vi "doRabi.vi"(8 "q_samples":i32=50, 9 "MW_Parameters":T1, 10 "parameters_recenter":T4={"input_xyz"={"X_um"=0.0, "Y_um"=0.0, "Z_um"=0.0}, "recenter"=FALSE, "recenter_s"=3}, 11 "Rabi_parameters":T5) -> (0 "triggers":u32[][](array[numeric]), 1 "std_deviation":dbl[](array[numeric]), 2 "Rabi_curve":cluster{dbl[], "dark_time_us":dbl[]}(graph), 3 "timetags":u32[][](array[numeric]))   [LabVIEW 2018]
uses:
  <vilib>/Analysis/NI_AALBase.lvlib
  <instrlib>/Rohde&Schwarz RF Signal Generator/Rohde&Schwarz RF Signal Generator.lvlib
panel:
  in  "parameters_z-scan":T2={"dwell_time_ms"=2.0, "q_steps"=5, "span_um"=1.0, "refocus"=TRUE}
  in  "parameters_xy-scan":T3={"image_size_xy_um"=2.0, "frame_size_xy_px"=7, "dwell_time_ms"=0.5}
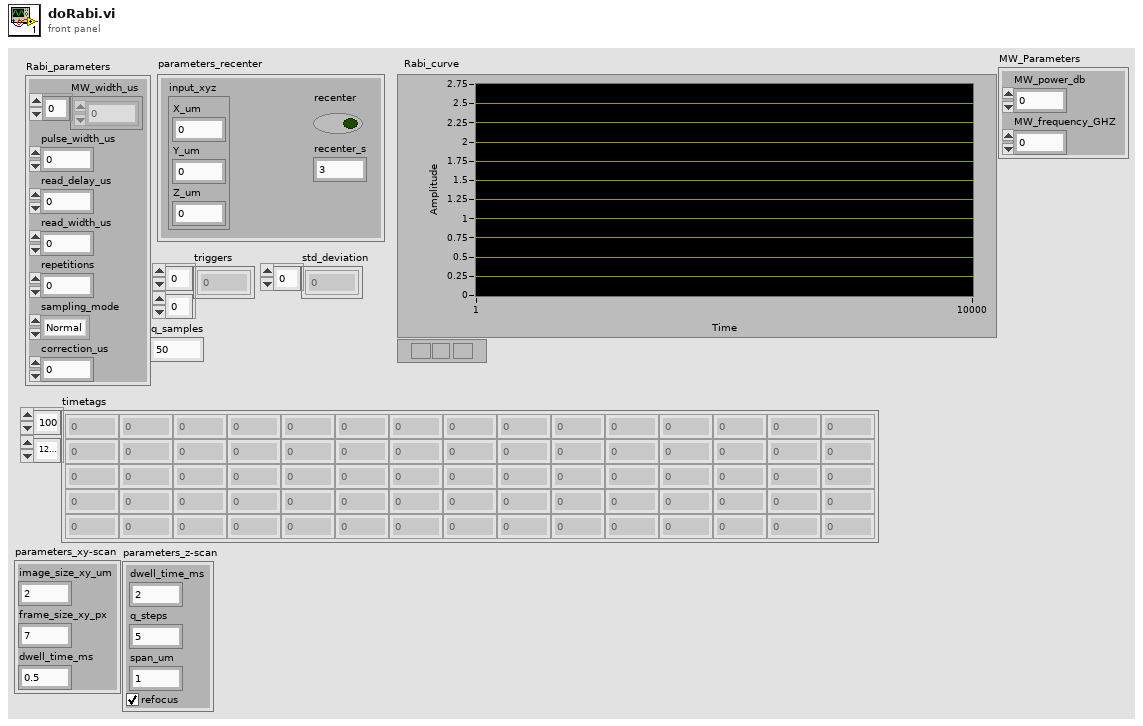
[diagram p1: front panel]
types:
  T1 = cluster{"MW_power_db":dbl, "MW_frequency_GHZ":dbl}
  T2 = cluster{"dwell_time_ms":dbl, "q_steps":u32, "span_um":dbl, "refocus":bool}
  T3 = cluster{"image_size_xy_um":dbl, "frame_size_xy_px":u32, "dwell_time_ms":dbl}
  T4 = cluster{"input_xyz":cluster{"X_um":sgl, "Y_um":sgl, "Z_um":sgl}, "recenter":bool, "recenter_s":u32}
  T5 = cluster{"MW_width_us":dbl[], "pulse_width_us":dbl, "read_delay_us":dbl, "read_width_us":dbl, "repetitions":i32, "sampling_mode":enum16{"Normal", "Sweep"}, "correction_us":dbl}
  T6 = cluster{"file_path":path, "file_name":string, "image":dbl[][][], "image_size_xy":cluster{"image_size_x_um":sgl, "image_size_y_um":sgl}, "pixel_dwell_time_ms":sgl, "Laser_power_mW":sgl, "pixel_size":dbl, "tile_ij":cluster{"tile_i":i32, "tile_j":i32}, "Objective":string, "ColorMarkers":cluster{dbl, u32}[], "timestamp":timestamp, "micro-position-xyz":cluster{"micro-position_x_mm":sgl, "micro-position_y_mm":sgl, "micro-position_z_mm":sgl}, "zero_xyz":cluster{"zero_x_mm":dbl, "zero_y_mm":dbl, "zero_z_mm":dbl}, "nano-position-xyz":cluster{"nano-position_x_V":sgl, "nano-position_y_V":sgl, "nano-position_z_V":sgl}, "Kxyz":cluster{"Kx_V/um":sgl, "Ky_V/um":sgl, "Kz_V/um":sgl}}
  T7 = cluster{"x_um":sgl[], "y_um":sgl[], "z_um":sgl[], "timetag":timestamp[]}
  T8 = cluster{"Instruct Data":i32, "Op Code":i32, "Flags":bool[], "Comments":string, "Time":dbl}[]
  T9 = cluster{"nano-position_X_um":sgl, "nano-position_Y_um":sgl, "nano-position Z_um":sgl}
  T10 = cluster{"nano-position_X_um":sgl, "nano-position_Y_um":sgl, "nano-position Z_um":sgl}[]
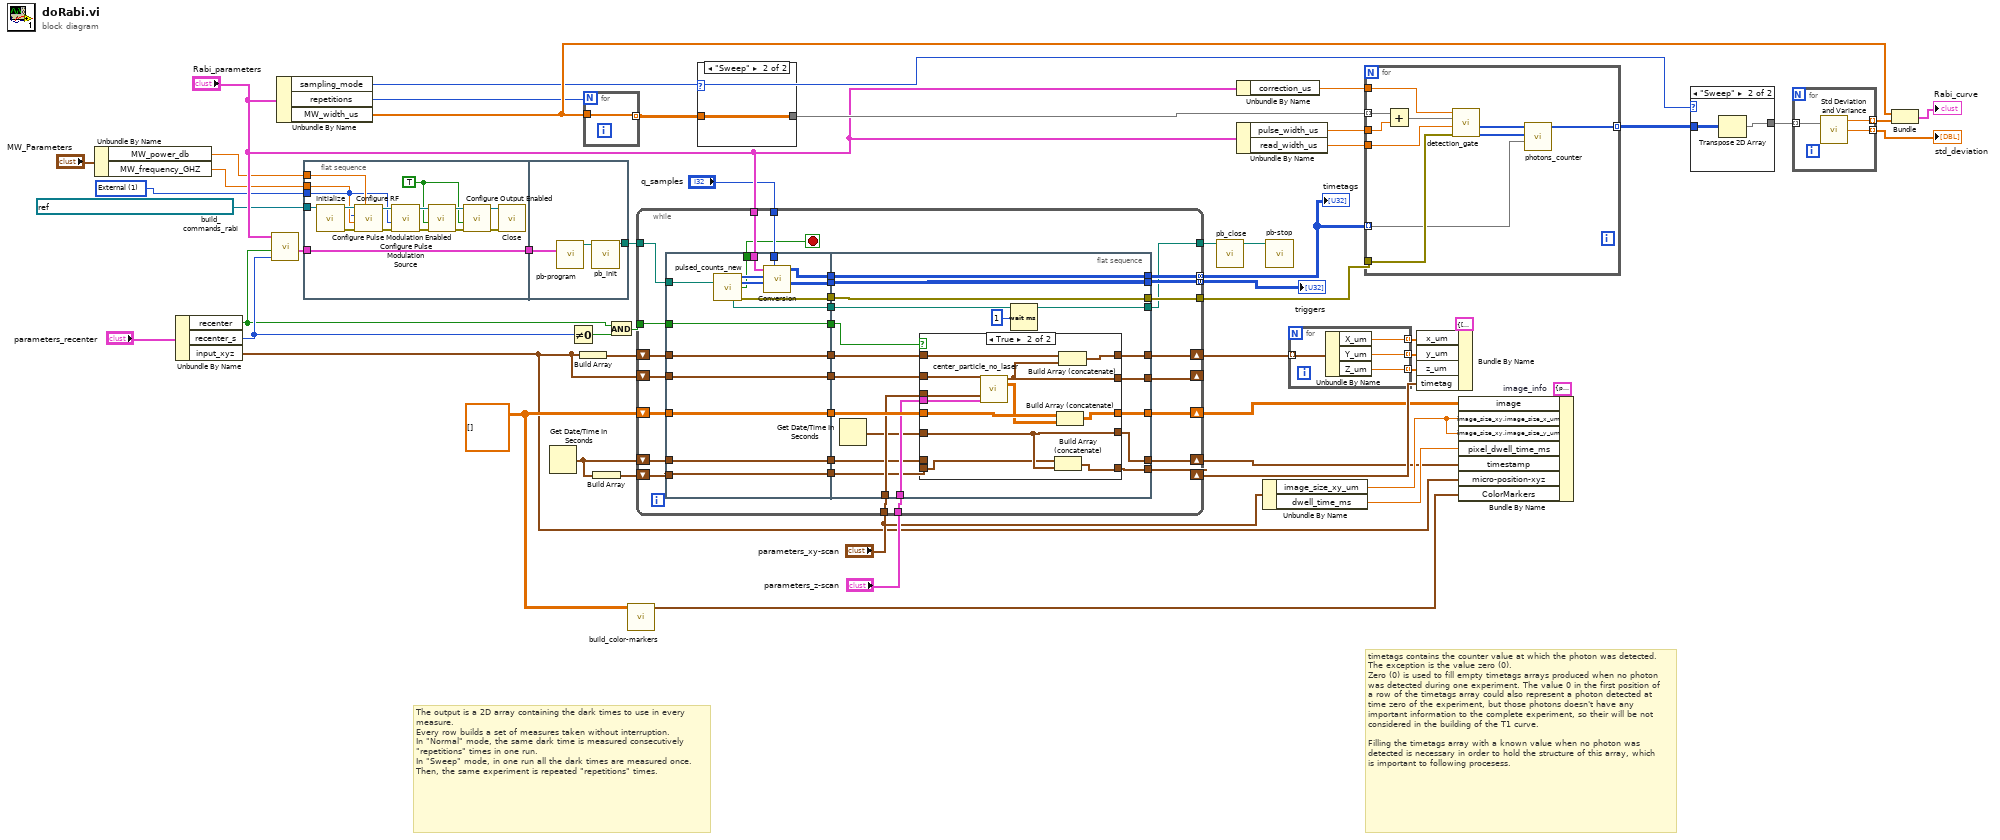
[diagram p0: block diagram]
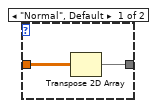
[diagram p3: hidden frame]
diagram:
  w1 = 1 items=["Auto", "External", "External Gated"] ("Trigger Mode (Auto)")
  w23 = T6 {"file_path"=path "", "file_name"="", "image"=[], "image_size_xy"={"image_size_x_um"=1.0, "image_size_y_um"=1.0}, "pixel_dwell_time_ms"=1.0, "Laser_power_mW"=1.0, "pixel_size"=0.0, "tile_ij"={"tile_i"=0, "tile_j"=0}, "Objective"="", "ColorMarkers"=[], "timestamp"=timestamp(0 s since 1904-01-01), "micro-position-xyz"={"micro-position_x_mm"=1.0, "micro-position_y_mm"=1.0, "micro-position_z_mm"=1.0}, "zero_xyz"={"zero_x_mm"=0.0, "zero_y_mm"=0.0, "zero_z_mm"=0.0}, "nano-position-xyz"={"nano-position_x_V"=1.0, "nano-position_y_V"=1.0, "nano-position_z_V"=1.0}, "Kxyz"={"Kx_V/um"=1.0, "Ky_V/um"=1.0, "Kz_V/um"=1.0}}  # image_info
  w34 = dbl[][][] []
  # "timetags contains the counter value at which the photon was detected. The exception is the value zero (0).\nZero (0) is used to fill empty timetags arrays produced when no photon was detected during one experiment. The value 0 in the first position of a row of the timetags array could also represent a photon detected at time zero of the experiment, but those photons doesn't have any important information to the complete experiment, so their will be not considered in the building of the T1 curve.\n\nFilling the timetags array with a known value when no photon was detected is necessary in order to hold the structure of this array, which is important to following procesess."
  # "The output is a 2D array containing the dark times to use in every measure.\nEvery row builds a set of measures taken without interruption.\nIn \"Normal\" mode, the same dark time is measured consecutively \"repetitions\" times in one run.\nIn \"Sweep\" mode, in one run all the dark times are measured once. Then, the same experiment is repeated \"repetitions\" times."
  n1 = Unbundle By Name("MW_Parameters") -> ("MW_power_db"=w3:dbl, "MW_frequency_GHZ"=w2:dbl)
  n2 = Unbundle By Name("parameters_recenter") -> ("recenter"=w14:bool, "recenter_s"=w36:u32, "input_xyz"=w18:cluster{"X_um":sgl, "Y_um":sgl, "Z_um":sgl})
  n3 = call "build_commands_rabi.vi"("Refocus_s"=w36, "Refocus?"=w14, "Rabi_parameters"="Rabi_parameters") -> ("commands"=w6:T8)  [unwired: 8 in]
  n4 = Unbundle By Name("Rabi_parameters") -> ("sampling_mode"=w43:enum16{"Normal", "Sweep"}, "repetitions"=w12:i32, "MW_width_us"=w44:dbl[])
  n5 = flat-sequence {
    tunnel: refnum<visa-resource-name> "USB0::0x0AAD::0x005F::262159::INSTR" ("VISA resource name") -> [w68]
    tunnel: w6 -> [w67]
    tunnel: [w67] -> w5
    tunnel: w3 -> [w56]
    tunnel: w2 -> [w55]
    tunnel: w1 -> [w54]
    tunnel: [w70] -> w8
    tunnel: w5 -> [w69]
    frame #0 {
      w53 = TRUE ("Pulse Modulation Enabled (Off)")
      n6 = call <instrlib>:"Initialize.vi"("VISA resource name"=w68) -> ("VISA resource name out"=w66:refnum<visa-resource-name>, "error out"=w61:errorcluster)  [unwired: 13 in]
      n7 = call <instrlib>:"Configure RF.vi"("Power Level (-30.0)"=w56, "error in (no error)"=w61, "Frequency (1GHz)"=w55, "Path (1)"=w54, "VISA resource name"=w66) -> ("error out"=w60:errorcluster, "VISA resource name out"=w65:refnum<visa-resource-name>)  [unwired: 5 in]
      n8 = call <instrlib>:"Configure Pulse Modulation Source.vi"("error in (no error)"=w60, "Source (Internal)"=w54, "VISA resource name"=w65) -> ("error out"=w59:errorcluster, "VISA resource name out"=w64:refnum<visa-resource-name>)  [unwired: 7 in]
      n9 = call <instrlib>:"Configure Pulse Modulation Enabled.vi"("error in (no error)"=w59, "Pulse Modulation Enabled (Off)"=w53, "VISA resource name"=w64) -> ("error out"=w58:errorcluster, "VISA resource name out"=w63:refnum<visa-resource-name>)  [unwired: 7 in]
      n10 = call <instrlib>:"Configure Output Enabled.vi"("error in (no error)"=w58, "Output Enabled (Off)"=w53, "VISA resource name"=w63) -> ("error out"=w57:errorcluster, "VISA resource name out"=w62:refnum<visa-resource-name>)  [unwired: 7 in]
      n11 = call <instrlib>:"Close.vi"("error in (no error)"=w57, "VISA resource name"=w62) -> ()  [unwired: 9 in, 1 out]
    }
    frame #1 {
      n12 = call "pb-program.vi"("Commands"=w69) -> ("path out"=w71:path)  [unwired: 10 in]
      n13 = call "pb_init.vi"("path in"=w71) -> ("path out"=w70:path)  [unwired: 9 in, 1 out]
    }
  }
  n14 = Get Date/Time In Seconds() -> (seconds since 1Jan1904=w31:timestamp)
  n15 = Not Equal To 0?(x=w36) -> (x != 0?=w37:bool)
  n16 = Build Array(w18) -> (w38:cluster{"X_um":sgl, "Y_um":sgl, "Z_um":sgl}[])
  n17 = for {
    N: w12 -> [_]
    tunnel: [w72] -> w42 mode=indexing
    tunnel: w44 -> [w72]
  }
  n18 = Build Array(w31) -> (w32:timestamp[])
  n19 = And(x=w14, y=w37) -> (x .and. y?=w35:bool)
  n20 = call "build_color-markers.vi"("images"=w34) -> ("color_markers"=w17:cluster{dbl, u32}[])  [unwired: 10 in]
  n21 = while {
    tunnel: [w103] -> w39
    tunnel: [w102] -> w15 mode=concatenating
    tunnel: [w101] -> w16 mode=concatenating
    shift-right: [w90] -> w30
    shift-left: w38 -> [w97]
    tunnel: w35 -> [w94]
    shift-right: [w91] -> _
    shift-left: w18 -> [w93]
    shift-right: [w79] -> w22
    shift-left: w34 -> [w89]
    tunnel: "parameters_xy-scan" -> [w87]
    tunnel: "parameters_z-scan" -> [w86]
    shift-right: [w80] -> w25
    shift-left: w32 -> [w85]
    shift-right: [w84] -> w19
    shift-left: w31 -> [w83]
    tunnel: "Rabi_parameters" -> [w78]
    tunnel: "q_samples" -> [w77]
    tunnel: w8 -> [w75]
    tunnel: [w73] -> w10
    stop <- w76 stop-if-true
    n22 = flat-sequence {
      tunnel: [w119] -> w100
      tunnel: [w112] -> w99
      tunnel: [w111] -> w98
      tunnel: w97 -> [w118]
      tunnel: [w118] -> w96
      tunnel: [w117] -> w95
      tunnel: w94 -> [w117]
      tunnel: w93 -> [w116]
      tunnel: [w116] -> w92
      tunnel: w89 -> [w115]
      tunnel: [w115] -> w88
      tunnel: w85 -> [w113]
      tunnel: w83 -> [w114]
      tunnel: [w114] -> w82
      tunnel: [w113] -> w81
      tunnel: w78 -> [w110]
      tunnel: w77 -> [w107]
      tunnel: [w106] -> w76
      tunnel: w75 -> [w105]
      tunnel: [w104] -> w74
      tunnel: [w136] -> w101
      tunnel: [w137] -> w102
      tunnel: [w138] -> w103
      tunnel: w100 -> [w138]
      tunnel: w99 -> [w137]
      tunnel: w98 -> [w136]
      tunnel: w96 -> [w135]
      tunnel: w95 -> [w120]
      tunnel: w92 -> [w134]
      tunnel: [w133] -> w91
      tunnel: [w132] -> w90
      tunnel: w88 -> [w131]
      tunnel: w87 -> [w130]
      tunnel: w86 -> [w129]
      tunnel: [w127] -> w84
      tunnel: w82 -> [w126]
      tunnel: w81 -> [w125]
      tunnel: [w124] -> w80
      tunnel: [w123] -> w79
      tunnel: w74 -> [w122]
      tunnel: [w122] -> w73
      frame #0 {
        n23 = call "pulsed_counts_new.vi"("path in"=w105) -> ("timetags"=w109:u32[], "triggers"=w108:u32[], "stop measure"=w106:bool, "path out"=w104:path, "Error_out"=w119:errorcluster)  [unwired: 10 in]
        n24 = call "Conversion.vi"("q_samples"=w107, "triggers"=w108, "timetags"=w109, "Rabi_parameters"=w110) -> ("triggers"=w112:u32[][], "timetags"=w111:u32[][])  [unwired: 6 in]
      }
      frame #1 {
        n25 = Get Date/Time In Seconds() -> (seconds since 1Jan1904=w128:timestamp)
        n26 = case shown="True" w120 {
          tunnel: w135 -> [w143 w155]
          tunnel: w134 -> [w142 w154]
          tunnel: [w142 w153] -> w133
          tunnel: [w143 w152] -> w132
          tunnel: w131 -> [w139 w151]
          tunnel: w130 -> [_ w149]
          tunnel: w129 -> [_ w148]
          tunnel: w128 -> [_ w147]
          tunnel: [w141 w147] -> w127
          tunnel: w126 -> [w141 _]
          tunnel: w125 -> [w140 w146]
          tunnel: [w140 w145] -> w124
          tunnel: [w139 w144] -> w123
          frame False {
          }
          frame True {
            n27 = call "center_particle_no_laser.vi"("input_xyz"=w154, "parameters_xy-scan"=w149, "parameters_z-scan"=w148) -> ("output_xyz"=w153:T9, "mini_scan"=w150:dbl[][])  [unwired: 11 in]
            n28 = Build Array (concatenate)(w146, w147) -> (w145:timestamp[])
            n29 = Build Array (concatenate)(w151, w150) -> (w144:dbl[][][])
            n30 = Build Array (concatenate)(w155, w153) -> (w152:T10)
          }
        }
        n31 = Wait (ms)(milliseconds to wait=u32 1) -> ()  [unwired: 1 out]
      }
    }
  }
  "timetags" <- w16
  "triggers" <- w15
  n32 = case shown="\"Sweep\"" w43 {
    tunnel: w42 -> [w157 w158]
    tunnel: [w156 w158] -> w41
    frame "Normal", Default {
      n33 = Transpose 2D Array(2D array=w157) -> (transposed array=w156:dbl[][])
    }
    frame "Sweep" {
    }
  }
  n34 = call "pb_close.vi"("path in"=w10) -> ("path out"=w9:path)  [unwired: 9 in, 1 out]
  n35 = Unbundle By Name("Rabi_parameters") -> ("correction_us"=w46:dbl)
  n36 = Unbundle By Name("Rabi_parameters") -> ("pulse_width_us"=w45:dbl, "read_width_us"=w47:dbl)
  n37 = Unbundle By Name("parameters_xy-scan") -> ("image_size_xy_um"=w21:dbl, "dwell_time_ms"=w20:dbl)
  n38 = call "pb-stop.vi"("path in"=w9) -> ()  [unwired: 9 in, 2 out]
  n39 = for {
    tunnel: w30 -> [w162] mode=indexing
    tunnel: [w161] -> w28 mode=indexing
    tunnel: [w160] -> w27 mode=indexing
    tunnel: [w159] -> w26 mode=indexing
    n40 = Unbundle By Name(w162) -> ("X_um"=w161:sgl, "Y_um"=w160:sgl, "Z_um"=w159:sgl)
  }
  n41 = for {
    tunnel: [w172] -> w48 mode=indexing
    tunnel: w47 -> [w171]
    tunnel: w39 -> [w170]
    tunnel: w46 -> [w167]
    tunnel: w45 -> [w166]
    tunnel: w41 -> [w164] mode=indexing
    tunnel: w16 -> [w163] mode=indexing
    n42 = Add(x=w164, y=w166) -> (x+y=w165:dbl[])
    n43 = call "detection_gate.vi"("Error_in"=w170, "read_width_us"=w171, "pulse_period_us"=w165, "correction_us"=w167) -> ("start_read"=w168:u32[], "stop_read"=w169:u32[])  [unwired: 6 in]
    n44 = call "photons_counter.vi"("timetags"=w163, "start_read"=w168, "stop_read"=w169) -> ("photons_counts"=w172:i32[])  [unwired: 8 in]
  }
  n45 = Bundle By Name(cluster=T7 {"x_um"=[], "y_um"=[], "z_um"=[], "timetag"=[]} ("position_xyzt"), "x_um"=w28, "y_um"=w27, "z_um"=w26, "timetag"=w25) -> ()  [unwired: 1 out]
  n46 = Bundle By Name(cluster=w23, "image"=w22, "image_size_xy.image_size_x_um"=w21, "image_size_xy.image_size_y_um"=w21, "pixel_dwell_time_ms"=w20, "timestamp"=w19, "micro-position-xyz"=w18, "ColorMarkers"=w17) -> ()  [unwired: 1 out]
  n47 = case shown="\"Sweep\"" w43 {
    tunnel: w48 -> [w173 w175]
    tunnel: [w173 w174] -> w51
    frame "Normal", Default {
    }
    frame "Sweep" {
      n48 = Transpose 2D Array(2D array=w175) -> (transposed array=w174:i32[][])
    }
  }
  n49 = for {
    tunnel: w51 -> [w178] mode=indexing
    tunnel: [w177] -> w50 mode=indexing
    tunnel: [w176] -> w49 mode=indexing
    n50 = call <vilib>:"Std Deviation and Variance.vi"("X"=w178) -> ("mean"=w177:dbl, "standard deviation"=w176:dbl)  [unwired: 1 in, 1 out]
  }
  "std_deviation" <- w49
  n51 = Bundle("MW_width_us"=w44, w50) -> (→"Rabi_curve":cluster{"MW_width_us":dbl[], dbl[]})  [unwired: 1 in]
